vi "RNG Create.vi"(8 "error in":errorcluster, 11 "State":u64) -> (0 "error out":errorcluster, 3 "RNG":refnum<class "RNG.lvclass">)   [LabVIEW 2020, in "OpenLvVision_OpenCv.lvlib" / "RNG.lvclass"]
doc: "Object by reference !\nThese are the RNG constructors. The first form sets the state to some pre-defined value, equal to 2**32-1 in the current implementation. The second form sets the state to the specified value. If you passed state=0 , the constructor uses the above default value instead to avoid the singular random number sequence, consisting of all zeros."
uses:
  RNG.lvclass
  _LvHelpers/EdvrObject/EdvrObject.lvclass
  OpenLvVision_OpenCv.lvlib
  _LvHelpers/EdvrObject/TypeDef/Edvr.ctl
  Dlls/OlvOpenCvWrapper.dll
  C:/Users/lukas/Downloads/OpenLvVision_OpenCv/SourceCode/LabView/OpenLvVision_OpenCv/_LvHelpers/EdvrObject/EdvrObject.lvclass
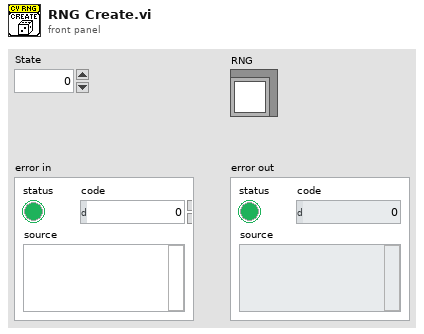
[diagram p1: front panel]
types:
  T1 = typedef "OpenLvVision_OpenCv.lvlib/EdvrObject.lvclass/Edvr.ctl" = refnum<data-value>
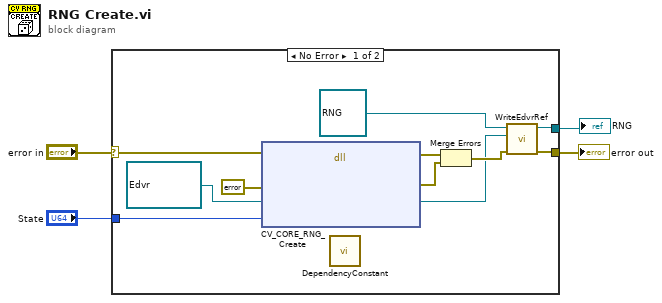
[diagram p0: block diagram]
diagram:
  n1 = case shown="No Error" "error in" {
    selector: "error in" -> [w11 w16]
    tunnel: [w14 w16] -> w3
    tunnel: [w15 _] -> w2
    tunnel: "State" -> [w10 _]
    frame No Error {
      n2 = dll-call lib="C:/Users/lukas/Downloads/OpenLvVision_OpenCv/SourceCode/LabView/OpenLvVision_OpenCv/Dlls/OlvOpenCvWrapper.dll" fn="CV_CORE_RNG_Create"(error in=w11, "Error"=errorcluster {"status"=FALSE, "code"=0, "source"=""} ("error out"), "edvrRef"=T1 refnum ("Edvr"), "state"=w10) -> (error out=w8:errorcluster, "Error"=w5:errorcluster, "edvrRef"=w6:T1)  [unwired: 4 in, 1 out]
      n3 = call "DependencyConstant.vi"() -> ()  [unwired: 12 in]
      n4 = Merge Errors(w8, w5) -> (w7:errorcluster)
      n5 = call "WriteEdvrRef.vi"("error in (no error)"=w7, "Edvr"=w6, "EdvrObject in"=refnum<class "RNG.lvclass"> refnum ("OpenLvVision_OpenCv.lvlib:RNG")) -> ("error out"=w14:errorcluster, "EdvrObject out"=w15:refnum<class "RNG.lvclass">)  [unwired: 7 in]
    }
    frame Error {
    }
  }
  "RNG" <- w2
  "error out" <- w3
